vi "Color_HighlightDescription.vi"(11 "String in":refnum<vi>) -> (3 "String out":refnum<vi>)   [LabVIEW 2022 SP3]
uses:
  Color_Globals.vi
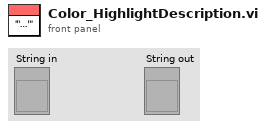
[diagram p1: front panel]
types:
  T1 = cluster{"offset past match":i32, "offset past match":i32}
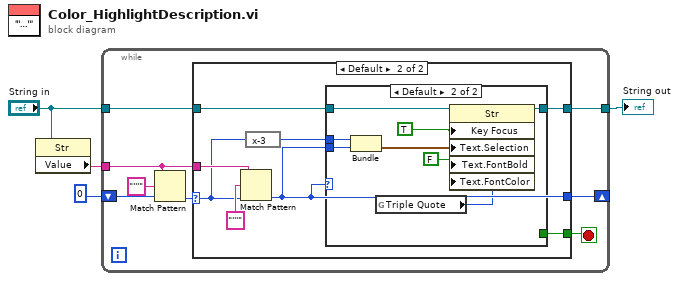
[diagram p0: block diagram]
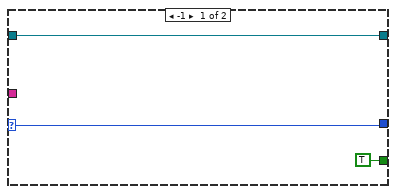
[diagram p2: hidden frame]
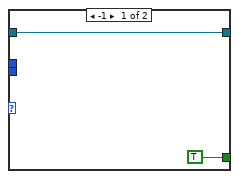
[diagram p3: hidden frame]
diagram:
  n1 = property on="Property Node" class="Str"(reference="String in") -> ("Value"=w1:string)  [unwired: 1 in, 2 out]
  n2 = while {
    tunnel: w1 -> [w8]
    shift-right: [w10] -> _
    shift-left: 0 -> [w12]
    tunnel: "String in" -> [w9]
    tunnel: [w7] -> w4
    stop <- w5 stop-if-true
    n3 = Match Pattern(string=w8, regular expression="'''", offset (0)=w12) -> (offset past match=w6:i32)  [unwired: 3 out]
    n4 = case shown="Default" w6 {
      selector: w6 -> [w14 w17]
      tunnel: [w14 w19] -> w10
      tunnel: w9 -> [w15 w22]
      tunnel: w8 -> [_ w21]
      tunnel: [w15 w20] -> w7
      tunnel: [TRUE w18] -> w5
      frame -1 {
      }
      frame Default {
        n5 = Match Pattern(string=w21, regular expression="'''", offset (0)=w17) -> (offset past match=w19:i32)  [unwired: 3 out]
        n6 = expression code="x-3"(w17) -> (w16:i32)
        n7 = case shown="Default" w19 {
          tunnel: w19 -> [_ w33]
          tunnel: w22 -> [w24 w30]
          tunnel: w16 -> [_ w28]
          tunnel: [w24 w27] -> w20
          tunnel: [TRUE _] -> w18
          frame -1 {
          }
          frame Default {
            n8 = Bundle("offset past match"=w28, "offset past match"=w33) -> (w29:T1)  [unwired: 1 in]
            n9 = global read "Color_Globals.vi" "Triple Quote"() -> (w26:u32)
            n10 = property on="Property Node" class="Str"(reference=w30, "Key Focus"=TRUE, "Text.Selection"=w29, "Text.FontBold"=FALSE ("Text.Font:Bold"), "Text.FontColor"=w26) -> (reference out=w27:refnum<vi>)  [unwired: 1 in, 1 out]
          }
        }
      }
    }
  }
  "String out" <- w4
